vi "Test - Add to Definitions.vi"   [LabVIEW 2020, in "JSON Schema Generator.lvlib"]
uses:
  JSON Schema Generator.lvlib
  <vilib>/addons/_JKI Toolkits/Caraya/classes/Test/Test.lvclass
  <vilib>/addons/_JKI Toolkits/Caraya/classes/Assert/Assert.lvclass
  Defintion FGV Actions.ctl
  <vilib>/addons/_JKI Toolkits/Caraya/classes/Assert/Assert Not Error.vi
  <vilib>/addons/_JKI Toolkits/Caraya/classes/Assert/Assert Equal Value_Variant.vi
  16565a66-e069-4842-9075-a2a508ea047b.vi
types:
  T1 = typedef "JSON Schema Generator.lvlib/Defintion FGV Actions.ctl" = enum16{"Create Defs", "Update Defs", "Get all Defs", "Get Def"}
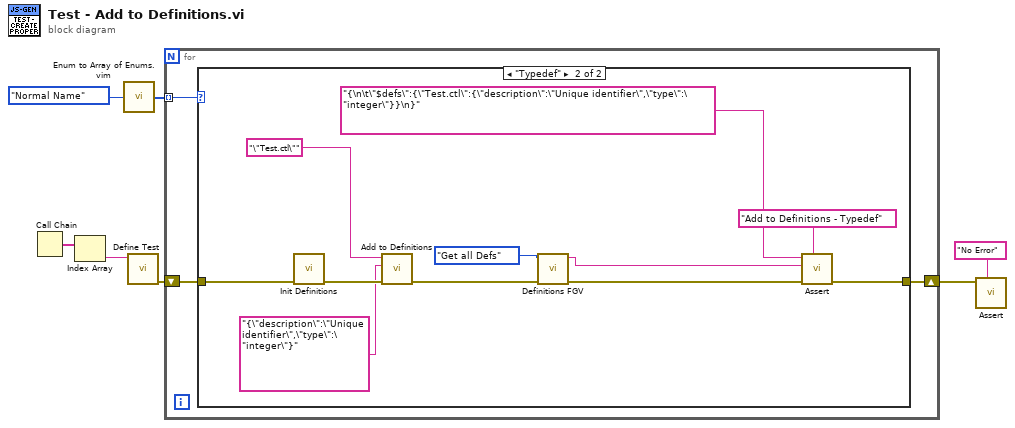
[diagram p0: block diagram]
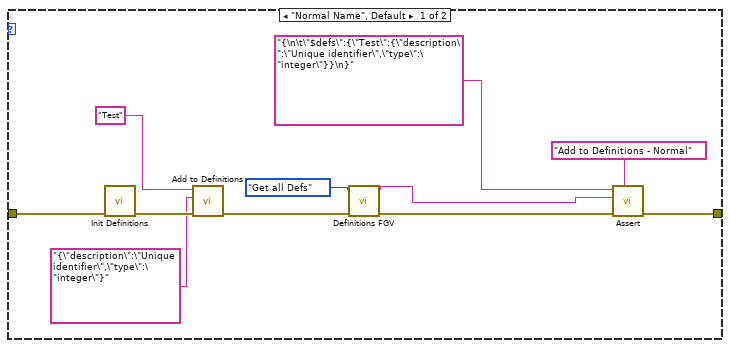
[diagram p2: hidden frame]
diagram:
  n1 = Call Chain() -> (call chain=w7:string[])
  n2 = Index Array(array=w7) -> (element=w6:string)  [unwired: 1 in]
  n3 = call "Enum to Array of Enums.vim"("enum"=enum16{"Normal Name", "Typedef"}."Normal Name") -> ("array of enums"=w1:enum16{"Normal Name", "Typedef"}[])
  n4 = call <vilib>:"Define Test.vi"("Label (VI Title)"=w6) -> ("error out"=w3:errorcluster)  [unwired: 9 in, 1 out]
  n5 = for {
    shift-right: [w9] -> w4
    shift-left: w3 -> [w10]
    tunnel: w1 -> [w8] mode=indexing
    n6 = case shown="\"Typedef\"" w8 {
      tunnel: [w21 w32] -> w9
      tunnel: w10 -> [w19 w30]
      frame "Normal Name", Default {
        n7 = call "Init Definitions.vi"("error in (no error)"=w19) -> ("error out (no error)"=w14:errorcluster)  [unwired: 10 in]
        n8 = call "Add to Definitions.vi"("error in (no error)"=w14, "Definition Schema"="{\"description\":\"Unique identifier\",\"type\":\"integer\"}", "Name"="Test") -> ("error out"=w13:errorcluster)  [unwired: 8 in]
        n9 = call "Definitions FGV.vi"("error in (no error)"=w13, "Action"=Defintion_FGV_Actions."Get all Defs") -> ("error out"=w17:errorcluster, "Definitions out"=w15:string)  [unwired: 7 in, 1 out]
        n10 = call-poly <vilib>:"Assert.vi"("Label"="Add to Definitions - Normal", "error in (no error)"=w17, "Actual"=w15, "Expected"="{\n\t\"$defs\":{\"Test\":{\"description\":\"Unique identifier\",\"type\":\"integer\"}}\n}") -> ("error out"=w21:errorcluster)  [unwired: 6 in, 1 out]
      }
      frame "Typedef" {
        n11 = call "Init Definitions.vi"("error in (no error)"=w30) -> ("error out (no error)"=w26:errorcluster)  [unwired: 10 in]
        n12 = call "Add to Definitions.vi"("error in (no error)"=w26, "Definition Schema"="{\"description\":\"Unique identifier\",\"type\":\"integer\"}", "Name"="\"Test.ctl\"") -> ("error out"=w25:errorcluster)  [unwired: 8 in]
        n13 = call "Definitions FGV.vi"("error in (no error)"=w25, "Action"=Defintion_FGV_Actions."Get all Defs") -> ("error out"=w28:errorcluster, "Definitions out"=w27:string)  [unwired: 7 in, 1 out]
        n14 = call-poly <vilib>:"Assert.vi"("Label"="Add to Definitions - Typedef", "error in (no error)"=w28, "Actual"=w27, "Expected"="{\n\t\"$defs\":{\"Test.ctl\":{\"description\":\"Unique identifier\",\"type\":\"integer\"}}\n}" ("JSON")) -> ("error out"=w32:errorcluster)  [unwired: 6 in, 1 out]
      }
    }
  }
  n15 = call-poly <vilib>:"Assert.vi"("Label"="No Error", "Not Error?"=w4) -> ()  [unwired: 8 in, 2 out]
